vi "createInterface.vi"(8 "error in (no error)":errorcluster, 11 "Orion_BMS in":refnum<class "Orion_BMS.lvclass">) -> (0 "error out":errorcluster, 2 "interface object out":refnum<k20>, 3 "Orion_BMS out":refnum<class "Orion_BMS.lvclass">)   [LabVIEW 2017, in "Orion_BMS.lvclass"]
uses:
  Orion_BMS.lvclass
  Orion_BMS.lvclass/Orion_BMS.ctl
  <vilib>/CANopenLib/CANOPEN.llb/CANopen Interface Create.vi
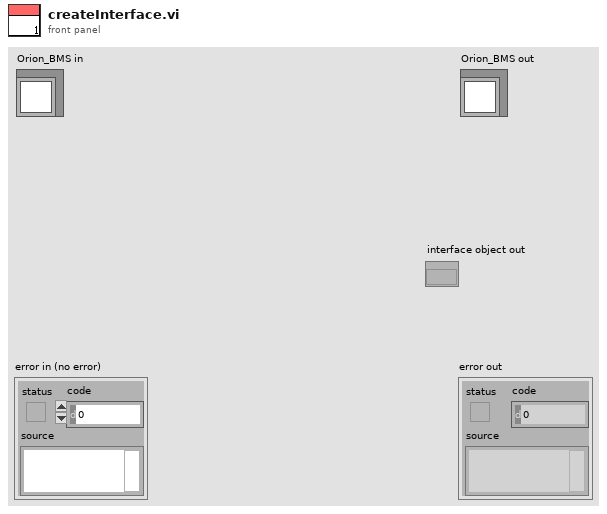
[diagram p1: front panel]
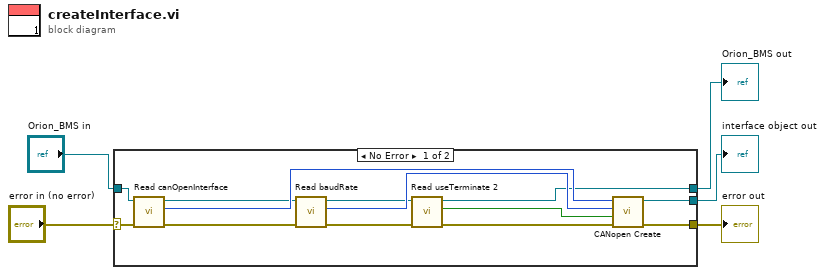
[diagram p0: block diagram]
diagram:
  n1 = case shown="No Error" "error in (no error)" {
    selector: "error in (no error)" -> [w14 w20]
    tunnel: [w15 w20] -> w4
    tunnel: [w8 w19] -> w2
    tunnel: "Orion_BMS in" -> [w18 w19]
    tunnel: [w16 _] -> w1
    frame No Error {
      n2 = call "Read canOpenInterface.vi"("error in (no error)"=w14, "OrionBMS in"=w18) -> ("error out"=w12:errorcluster, "canOpenInterface"=w17:u32, "OrionBMS out"=w13:refnum<class "Orion_BMS.lvclass">)  [unwired: 7 in]
      n3 = call "Read baudRate.vi"("error in (no error)"=w12, "OrionBMS in"=w13) -> ("error out"=w10:errorcluster, "baudRate"=w11:u32, "OrionBMS out"=w9:refnum<class "Orion_BMS.lvclass">)  [unwired: 7 in]
      n4 = call "Read useTerminate 2.vi"("error in (no error)"=w10, "Orion_BMS in"=w9) -> ("error out"=w6:errorcluster, "useTerminate"=w7:bool, "Orion_BMS out"=w8:refnum<class "Orion_BMS.lvclass">)  [unwired: 7 in]
      n5 = call-poly <vilib>:"CANopen Create.vi"("error in (no error)"=w6, "termination? (F)"=w7, "baud rate"=w11, "interface name"=w17) -> ("error out"=w15:errorcluster, "interface object out"=w16:refnum<k20>)  [unwired: 6 in]
    }
    frame Error {
    }
  }
  "error out" <- w4
  "Orion_BMS out" <- w2
  "interface object out" <- w1
